vi "Untitled 2.vi"() -> ()   [LabVIEW 2017]
uses:
  UI Error Handlers/support/Message Queue/Message Cluster.ctl
  Globals/Global - Configuration Options.vi
  UI Error Handlers/support/Message Queue/Message Queue.lvlib
panel:
  out "error out 2":errorcluster
  out "error out":errorcluster
  out "concatenated string":string
  out "resulting string 2":string
  out "reader name":string="UI Reader"
  in  "error in (no error)":errorcluster
  in  "Controller Address":string
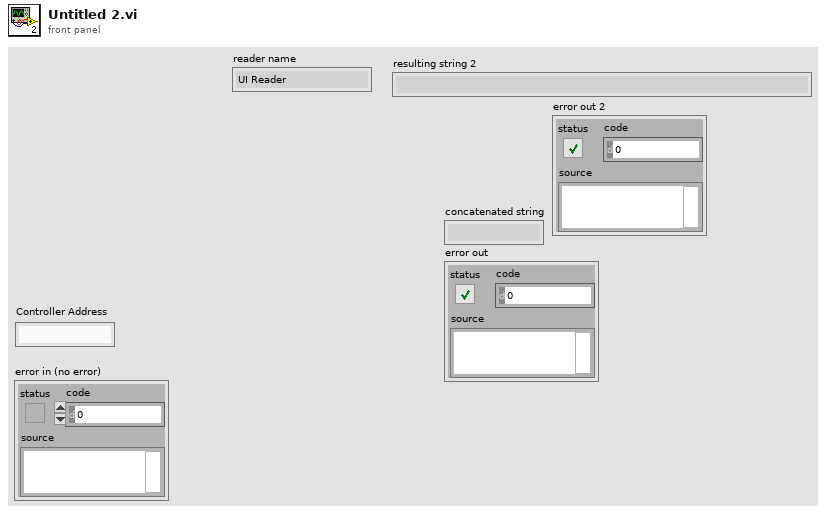
[diagram p1: front panel]
types:
  T1 = typedef "Message Queue.lvlib/Message Cluster.ctl" = cluster{"Message":string, "Message Data":variant}
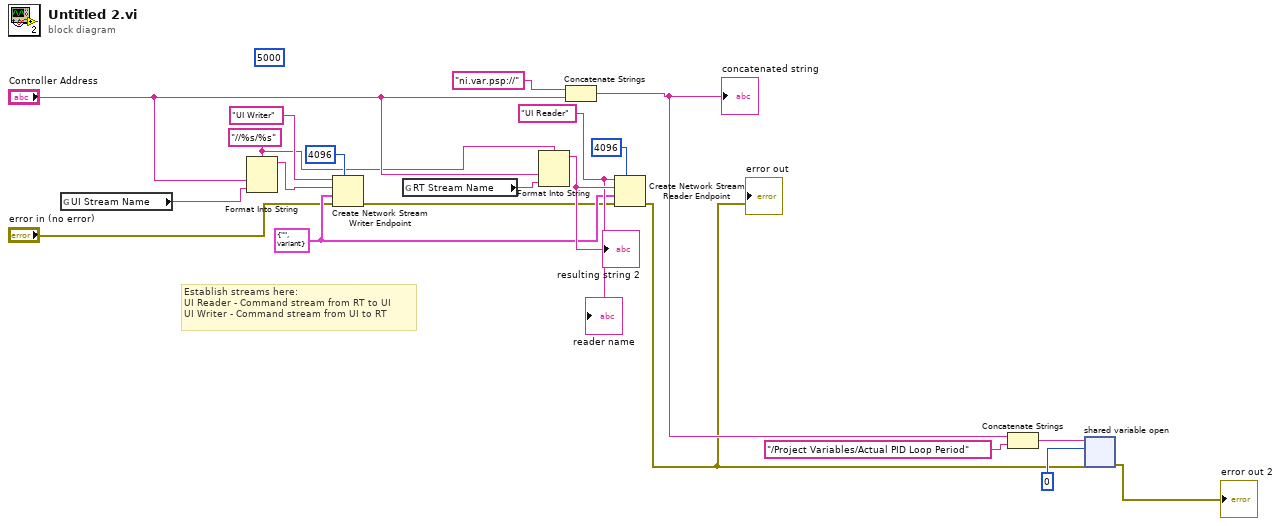
[diagram p0: block diagram]
diagram:
  (unwired) 5000 ("writer buffer size")
  w16 = T1 {"Message"="", "Message Data"=variant} ("Message Cluster")
  w17 = "UI Reader" ("reader name")
  w10 = "//%s/%s"
  # "Establish streams here:\nUI Reader - Command stream from RT to UI\nUI Writer - Command stream from UI to RT"
  n1 = global read "Global - Configuration Options.vi" "UI Stream Name"() -> (w9:string)
  n2 = Format Into String(format string=w10, "Controller Address", w9) -> (resulting string=w19:string)  [unwired: 2 in, 1 out]
  n3 = Create Network Stream Writer Endpoint(7:4096 ("writer buffer size"), 8:"error in (no error)", 9:w16, 10:w19, 11:"UI Writer" ("writer name")) -> (0:w7:errorcluster)  [unwired: 2 in, 1 out]
  n4 = global read "Global - Configuration Options.vi" "RT Stream Name"() -> (w8:string)
  n5 = Format Into String(format string=w10, "Controller Address", w8) -> (resulting string=w18:string)  [unwired: 2 in, 1 out]
  "resulting string 2" <- w18
  n6 = Concatenate Strings("ni.var.psp://", "Controller Address") -> (w3:string)
  "concatenated string" <- w3
  n7 = Create Network Stream Reader Endpoint(7:4096 ("reader buffer size"), 8:w7, 9:w16, 10:w18, 11:w17) -> (0:w2:errorcluster)  [unwired: 2 in, 1 out]
  "error out" <- w2
  n8 = Concatenate Strings(w3, "/Project Variables/Actual PID Loop Period") -> (w5:string)
  n9 = shared-variable-open(w5, w2, u32 0) -> (→"error out 2":errorcluster)  [unwired: 1 in, 1 out]
  "reader name" <- w17
